vi "Get Instance.vi"(8 "error in (no error)":errorcluster, 11 "Singleton":refnum<class "Singleton.lvclass">) -> (0 "error out":errorcluster, 3 "Instance Handle":T1)   [LabVIEW 2014, in "Singleton.lvclass"]
doc: "Obtains a reference to a session.\nIf session exists, vi returns active reference.\nIf session does not exist, vi runs 'set Defaults.vi' of session class hierarchy."
uses:
  Singleton.lvclass
  Typedefs/Instance handle.ctl
  Singleton.lvclass/Singleton.ctl
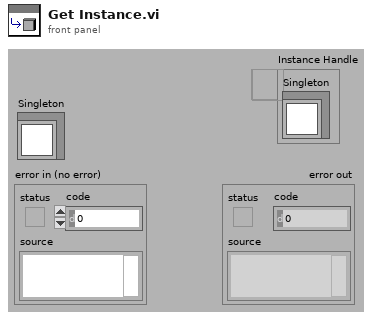
[diagram p1: front panel]
types:
  T1 = typedef "Singleton.lvclass/Instance handle.ctl" = refnum<data-value>
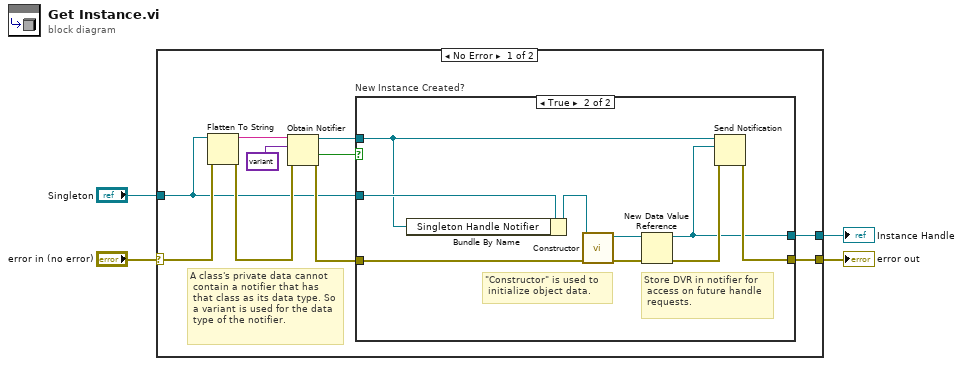
[diagram p0: block diagram]
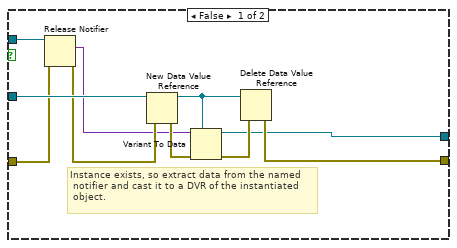
[diagram p2: hidden frame]
diagram:
  n1 = case shown="No Error" "error in (no error)" {
    selector: "error in (no error)" -> [w7 w34]
    tunnel: [w14 w34] -> w3
    tunnel: [w12 _] -> w2
    tunnel: "Singleton" -> [w5 _]
    frame No Error {
      # "A class's private data cannot\n contain a notifier that has\n that class as its data type. So\n a variant is used for the data\n type of the notifier."
      n2 = Flatten To String(anything=w5, error in (no error)=w7) -> (data string=w8:string, error out=w6:errorcluster)  [unwired: 2 in, 1 out]
      n3 = Obtain Notifier(name (unnamed)=w8, notification data type=variant ("Variant"), error in (no error)=w6) -> (notifier out=w11:refnum<notifier>, created new?=w13:bool, error out=w10:errorcluster)  [unwired: 1 in]
      n4 = case "New Instance Created?" shown="True" w13 {
        tunnel: w10 -> [w17 w25]
        tunnel: [w16 w33] -> w14
        tunnel: [w15 w31] -> w12
        tunnel: w11 -> [w18 w27]
        tunnel: w5 -> [w21 w28]
        frame False {
          # "Instance exists, so extract data from the named\n notifier and cast it to a DVR of the instantiated\n object."
          n5 = Release Notifier(notifier=w18, error in (no error)=w17) -> (last notification=w19:variant, error out=w20:errorcluster)  [unwired: 1 in, 1 out]
          n6 = New Data Value Reference(data value=w21, error in=w20) -> (data value reference=w24:refnum<data-value>, error out=w22:errorcluster)
          n7 = Variant To Data(error in=w22, type=w24, Variant=w19) -> (data=w15:refnum<data-value>, error out=w23:errorcluster)
          n8 = Delete Data Value Reference(data value reference=w24, error in=w23) -> (error out=w16:errorcluster)  [unwired: 1 out]
        }
        frame True {
          # "Store DVR in notifier for\n access on future handle\n requests."
          # "\"Constructor\" is used to\n initialize object data."
          n9 = Bundle By Name(cluster=w28, "Singleton Handle Notifier"=w27) -> (w26:refnum<class "Singleton.lvclass">)
          n10 = call-dynamic "Constructor.vi"("error in"=w25, "Singleton Abstract"=w26) -> ("error out"=w30:errorcluster, "Singleton Abstract"=w29:refnum<class "Singleton.lvclass">)  [unwired: 8 in]
          n11 = New Data Value Reference(data value=w29, error in=w30) -> (data value reference=w31:refnum<data-value>, error out=w32:errorcluster)
          n12 = Send Notification(notification=w31, notifier=w27, error in (no error)=w32) -> (error out=w33:errorcluster)  [unwired: 1 out]
        }
      }
    }
    frame Error {
    }
  }
  "error out" <- w3
  "Instance Handle" <- w2
